vi "define.vi"(8 "error in (no error)":errorcluster, 11 "TrajectoryAN1106117SinglePoint in":refnum<class "TrajectoryAN1106117SinglePoint.lvclass">) -> (0 "error out":errorcluster, 3 "TrajectoryAN1106117SinglePoint out":refnum<class "TrajectoryAN1106117SinglePoint.lvclass">)   [LabVIEW 2010, in "TrajectoryAN1106117SinglePoint.lvclass"]
doc: "modal dialog on which the user can set the trajectory parameters"
uses:
  TrajectoryAN1106117SinglePoint.lvclass
  common/xcontrols/XImage/XImage/XImage.xctl
  common/classes/ImageCollection/ImageCollection/ImageCollection.lvclass
  TrajectoryAN1106117SinglePoint.lvclass/TrajectoryAN1106117SinglePoint.ctl
panel:
  in  "cancelButton":bool
  in  "okButton":bool
  in  "Tab Control":enum32{"User", "About"}(tab)
  in  "XImage":refnum<class "ImageCollection.lvclass">(xcontrol)
  in  "number of pixels":i32=1 min=1 step=1
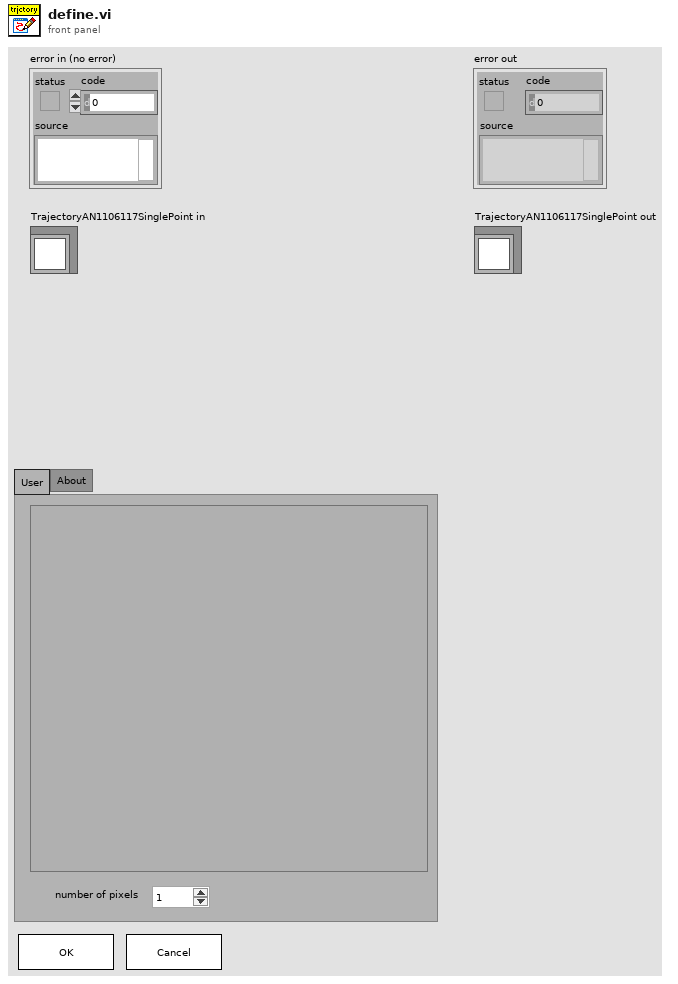
[diagram p1: front panel]
types:
  T1 = cluster{"Zoom Tool":bool, "Selection Tool":bool, "Pan Tool":bool, "Point Tool":bool, "Line Tool":bool, "Rectangle Tool":bool, "Rotated Rectangle Tool":bool, "Polyline Tool":bool, "Polygon Tool":bool, "Freehand Tool":bool, "Closed Freehand Tool":bool, "Ellipse Tool":bool, "Annulus Tool":bool}
  T2 = typedef "XImage.xctl/ROImicrons_frames_cluster.ctl" = cluster{"ROI":cluster{"Global Rectangle":dbl[unit][], "Contours":cluster{"Contour Type":u32, "ROI Type":u32, "Points":dbl[unit][]}[]}[]}
  T3 = cluster{"Global Rectangle":dbl[unit][], "Contours":cluster{"Contour Type":u32, "ROI Type":u32, "Points":dbl[unit][]}[]}[]
  T4 = cluster{"Global Rectangle":dbl[unit][], "Contours":cluster{"Contour Type":u32, "ROI Type":u32, "Points":dbl[unit][]}[]}
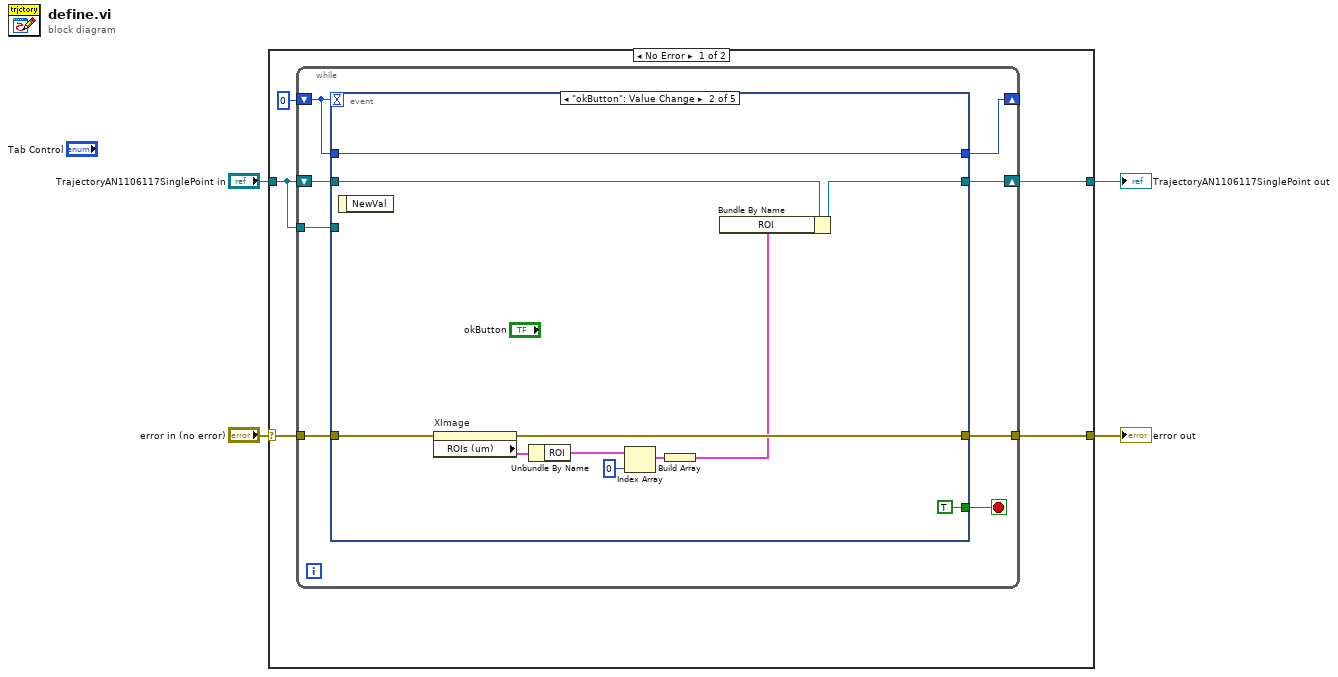
[diagram p0: block diagram]
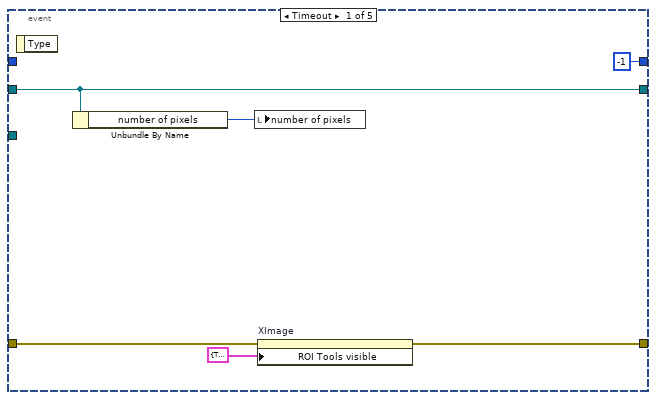
[diagram p2: hidden frame]
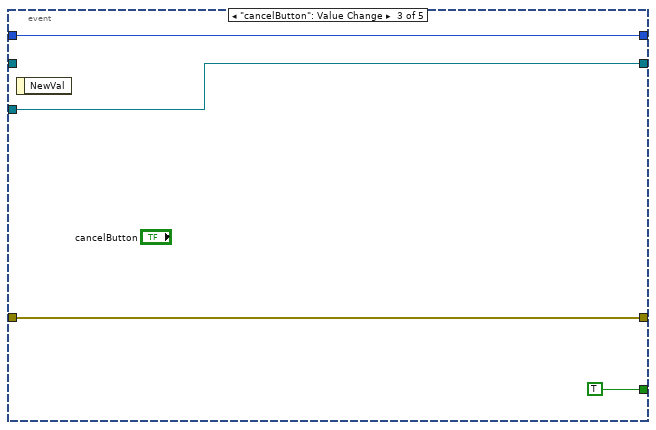
[diagram p3: hidden frame]
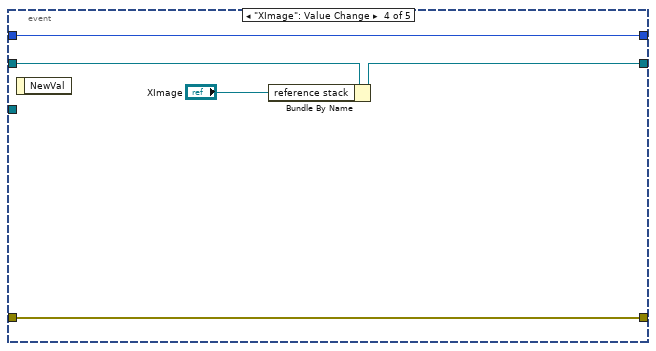
[diagram p4: hidden frame]
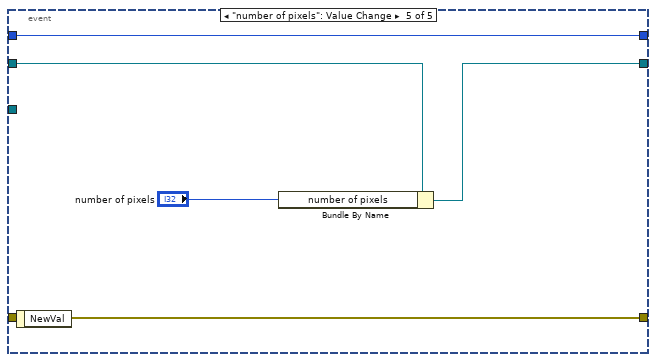
[diagram p5: hidden frame]
diagram:
  n1 = case shown="No Error" "error in (no error)" {
    selector: "error in (no error)" -> [w8 w50]
    tunnel: [w9 w50] -> w3
    tunnel: [w7 w49] -> w2
    tunnel: "TrajectoryAN1106117SinglePoint in" -> [w5 w49]
    frame No Error {
      n2 = while {
        tunnel: [w17] -> w9
        tunnel: w8 -> [w16]
        shift-right: [w13] -> _
        shift-left: 0 -> [w12]
        shift-right: [w15] -> w7
        shift-left: w5 -> [w14]
        tunnel: w5 -> [w10]
        stop <- w11 stop-if-true
        n3 = event shown="[1] \"okButton\": Value Change" {
          selector: _ -> [_ _ _ _ _]
          dyn-events: _ -> [_ _ _ _ _]
          timeout: w12 -> [_ _ _ _ _]
          tunnel: [w21 w31 w38 w43 w48] -> w17
          tunnel: w16 -> [w22 w32 w38 w43 w48]
          tunnel: [w19 w24 w35 w39 w46] -> w15
          tunnel: w14 -> [w19 w25 _ w40 w47]
          tunnel: [-1 w34 w37 w42 w44] -> w13
          tunnel: w12 -> [_ w34 w37 w42 w44]
          tunnel: [_ TRUE TRUE _ _] -> w11
          tunnel: w10 -> [_ _ w35 _ _]
          event Timeout {
            n4 = event-data() -> ()  [unwired: 1 in, 1 out]
            n5 = Unbundle By Name(w19) -> ("number of pixels"=w18:i32)
            n6 = local write "number of pixels"(w18) -> ()
            n7 = property on="XImage" class="XImage (strict)"(error in=w22, "ROI Tools visible"=T1 {"Zoom Tool"=TRUE, "Selection Tool"=TRUE, "Pan Tool"=TRUE, "Point Tool"=TRUE, "Line Tool"=FALSE, "Rectangle Tool"=FALSE, "Rotated Rectangle Tool"=FALSE, "Polyline Tool"=FALSE, "Polygon Tool"=FALSE, "Freehand Tool"=FALSE, "Closed Freehand Tool"=FALSE, "Ellipse Tool"=FALSE, "Annulus Tool"=FALSE} ("ROI:ROI Tools Palette visible")) -> (error out=w21:errorcluster)  [unwired: 1 in, 1 out]
          }
          event "okButton": Value Change {
            n8 = event-data() -> ()  [unwired: 1 in, 1 out]
            n9 = property on="XImage" class="XImage (strict)"(error in=w32) -> (error out=w31:errorcluster, "ROIs (um)"=w30:T2)  [unwired: 1 in, 1 out]
            n10 = Unbundle By Name(w30) -> ("ROI"=w29:T3)
            n11 = Index Array(array=w29, index=0) -> (element=w27:T4)
            n12 = Build Array(w27) -> (w26:T3)
            n13 = Bundle By Name(cluster=w25, "ROI"=w26) -> (w24:refnum<class "TrajectoryAN1106117SinglePoint.lvclass">)
          }
          event "cancelButton": Value Change {
            n14 = event-data() -> ()  [unwired: 1 in, 1 out]
          }
          event "XImage": Value Change {
            n15 = event-data() -> ()  [unwired: 1 in, 1 out]
            n16 = Bundle By Name(cluster=w40, "reference stack"="XImage") -> (w39:refnum<class "TrajectoryAN1106117SinglePoint.lvclass">)
          }
          event "number of pixels": Value Change {
            n17 = event-data() -> ()  [unwired: 1 in, 1 out]
            n18 = Bundle By Name(cluster=w47, "number of pixels"="number of pixels") -> (w46:refnum<class "TrajectoryAN1106117SinglePoint.lvclass">)
          }
        }
      }
    }
    frame Error {
    }
  }
  "error out" <- w3
  "TrajectoryAN1106117SinglePoint out" <- w2
